vi "Setup Hall Effect Library.vi"(8 "error in (no error)":errorcluster, 9 "Test Input Parameters":T8={"Current Level "=0.001, "Compliance Level"=1.0, "Soak Time"=0.0, "NPLC Voltmeter"=1.0, "Count Voltmeter"=1, "NPLC Ammeter"=1.0, "Count Ammeter"=1, "Sample Resistivity"=enum."Low", "Sample Thickness"=1.0, "Magnetic Flux"=0.57, "Units"=enum."T", "Sample Dimensions x"=0.0, "Sample Dimensions y"=0.0, "Sample Dimensions D1"=0.0, "Sample Dimensions D2"=0.0, "Sample Width Ws"=0.0, "Slot Number of 3765 Card"=0} {"NPLC Ammeter" min=0.01 max=10.0; "NPLC Voltmeter" min=0.01 max=10.0 format="%^#_6g"; "Count Ammeter" min=1 max=1024; "Count Voltmeter" min=1 max=1024; "Magnetic Flux" min=0.0; "Soak Time" min=0.0 format="%^#_6g"; "Sample Thickness" min=0.0; "Current Level" min=0.0 max=0.1 format="%^#_6e"; "Compliance Level" min=0.0 max=8.0 format="%^#_6g"}, 10 "Instrument Locations":T9, 11 "Instruments":T6={"Magnet"=enum."Manual", "Ammeter"=enum."648X", "Current Source"=enum."622X", "Switch"=enum."3706A", "Voltmeter"=enum."2182A"}) -> (0 "error out":errorcluster)   [LabVIEW 2016]
uses:
  Hall Effect Library/Public/Controls/Resisitivity.ctl
  Hall Effect Library/Public/Controls/Magnets.ctl
  Hall Effect Library/Public/Controls/Ammeters.ctl
  Hall Effect Library/Public/Controls/I-Sources.ctl
  Hall Effect Library/Public/Controls/Switches.ctl
  Hall Effect Library/Public/Controls/Voltmeters.ctl
  Hall Effect Library/Hall Effect Library.lvlib
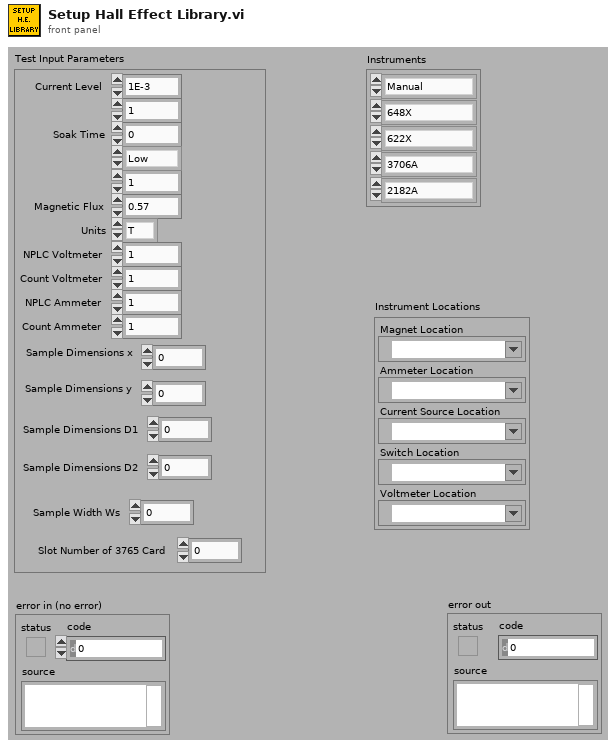
[diagram p1: front panel]
types:
  T1 = typedef "Hall Effect Library.lvlib/Magnets.ctl" = enum16{"Manual"}
  T2 = typedef "Hall Effect Library.lvlib/Ammeters.ctl" = enum16{"None", "648X"}
  T3 = typedef "Hall Effect Library.lvlib/I-Sources.ctl" = enum16{"622X", "26XX"}
  T4 = typedef "Hall Effect Library.lvlib/Switches.ctl" = enum16{"3706A"}
  T5 = typedef "Hall Effect Library.lvlib/Voltmeters.ctl" = enum16{"2000", "2182A", "3706A"}
  T6 = cluster{"Magnet":T1, "Ammeter":T2, "Current Source":T3, "Switch":T4, "Voltmeter":T5}
  T7 = typedef "Hall Effect Library.lvlib/Resisitivity.ctl" = enum16{"Low", "High"}
  T8 = cluster{"Current Level ":dbl, "Compliance Level":dbl, "Soak Time":dbl, "NPLC Voltmeter":dbl, "Count Voltmeter":i32, "NPLC Ammeter":dbl, "Count Ammeter":i32, "Sample Resistivity":T7, "Sample Thickness":dbl, "Magnetic Flux":dbl, "Units":enum16{"Gs", "T"}, "Sample Dimensions x":dbl, "Sample Dimensions y":dbl, "Sample Dimensions D1":dbl, "Sample Dimensions D2":dbl, "Sample Width Ws":dbl, "Slot Number of 3765 Card":u32}
  T9 = cluster{"Magnet Location":refnum<visa-resource-name>, "Ammeter Location":refnum<visa-resource-name>, "Current Source Location":refnum<visa-resource-name>, "Switch Location":refnum<visa-resource-name>, "Voltmeter Location":refnum<visa-resource-name>}
  T10 = cluster{"Resistivity":T7, "Compliance Level (Volts)":dbl, "Current Level (Amps)":dbl, "Soak Time (Seconds)":dbl, "Sample Thickness (cm)":dbl, "Magnetic Flux (Gauss)":dbl, "NPLC Ammeter":dbl, "Count Ammeter":i32, "NPLC Voltmeter":dbl, "Count Voltmeter":i32, "Sample Dimensions x":dbl, "Sample Dimensions y":dbl, "Sample Dimensions D1":dbl, "Sample Dimensions D2":dbl, "Sample Width Ws":dbl, "Slot Number of 3765 Card":u32}
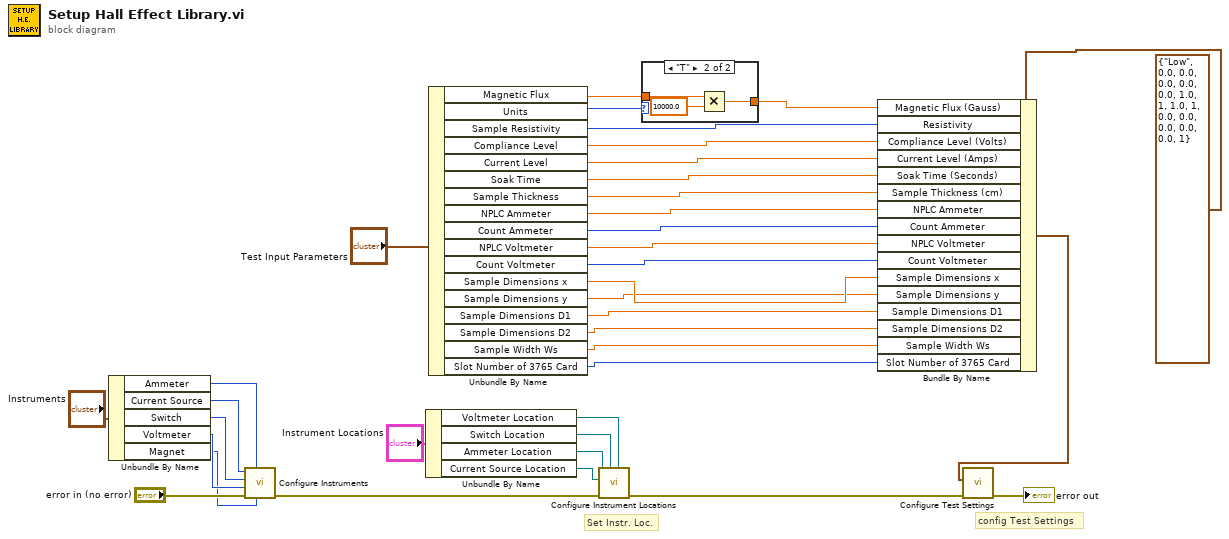
[diagram p0: block diagram]
diagram:
  # "config Test Settings"
  # "Set Instr. Loc."
  n1 = Unbundle By Name("Instruments") -> ("Ammeter"=w13:T2, "Current Source"=w12:T3, "Switch"=w11:T4, "Voltmeter"=w10:T5, "Magnet"=w6:T1)
  n2 = call "Configure Instruments.vi"("Magnet"=w6, "Ammeter"=w13, "error in (no error)"="error in (no error)", "Voltmeter"=w10, "Switch"=w11, "Current Source"=w12) -> ("error out"=w15:errorcluster)  [unwired: 5 out]
  n3 = Unbundle By Name("Instrument Locations") -> ("Voltmeter Location"=w35:refnum<visa-resource-name>, "Switch Location"=w36:refnum<visa-resource-name>, "Ammeter Location"=w30:refnum<visa-resource-name>, "Current Source Location"=w31:refnum<visa-resource-name>)
  n4 = Unbundle By Name("Test Input Parameters") -> ("Magnetic Flux"=w27:dbl, "Units"=w26:enum16{"Gs", "T"}, "Sample Resistivity"=w17:T7, "Compliance Level"=w18:dbl, "Current Level"=w19:dbl, "Soak Time"=w20:dbl, "Sample Thickness"=w21:dbl, "NPLC Ammeter"=w22:dbl, "Count Ammeter"=w23:i32, "NPLC Voltmeter"=w24:dbl, "Count Voltmeter"=w25:i32, "Sample Dimensions x"=w9:dbl, "Sample Dimensions y"=w8:dbl, "Sample Dimensions D1"=w7:dbl, "Sample Dimensions D2"=w3:dbl, "Sample Width Ws"=w2:dbl, "Slot Number of 3765 Card"=w1:u32)
  n5 = call "Configure Instrument Locations.vi"("V-Meter"=w35, "Switch"=w36, "error in (no error)"=w15, "I-SRC"=w31, "Ammeter"=w30) -> ("error out"=w33:errorcluster)  [unwired: 1 in, 5 out]
  n6 = case shown="\"T\"" w26 {
    tunnel: w27 -> [w37 w40]
    tunnel: [w37 w38] -> w28
    frame "Gs", Default {
    }
    frame "T" {
      n7 = Multiply(x=w40, y=10000.0) -> (x*y=w38:dbl)
    }
  }
  n8 = Bundle By Name(cluster=T10 {"Resistivity"=enum."Low", "Compliance Level (Volts)"=0.0, "Current Level (Amps)"=0.0, "Soak Time (Seconds)"=0.0, "Sample Thickness (cm)"=0.0, "Magnetic Flux (Gauss)"=0.0, "NPLC Ammeter"=1.0, "Count Ammeter"=1, "NPLC Voltmeter"=1.0, "Count Voltmeter"=1, "Sample Dimensions x"=0.0, "Sample Dimensions y"=0.0, "Sample Dimensions D1"=0.0, "Sample Dimensions D2"=0.0, "Sample Width Ws"=0.0, "Slot Number of 3765 Card"=1} ("Test Settings"), "Magnetic Flux (Gauss)"=w28, "Resistivity"=w17, "Compliance Level (Volts)"=w18, "Current Level (Amps)"=w19, "Soak Time (Seconds)"=w20, "Sample Thickness (cm)"=w21, "NPLC Ammeter"=w22, "Count Ammeter"=w23, "NPLC Voltmeter"=w24, "Count Voltmeter"=w25, "Sample Dimensions x"=w9, "Sample Dimensions y"=w8, "Sample Dimensions D1"=w7, "Sample Dimensions D2"=w3, "Sample Width Ws"=w2, "Slot Number of 3765 Card"=w1) -> (w4:T10)
  n9 = call "Configure Test Settings.vi"("error in (no error)"=w33, "Test Settings"=w4) -> ("error out"=→"error out":errorcluster)  [unwired: 5 in, 4 out]
